vi "__FilterSet_SelfDefine.vi"(8 "error in (no error)":errorcluster, 9 "EIDRef":refnum<vi>[](array[refnum]), 10 "IDRef":refnum<vi>[](array[refnum]), 11 "ControlRef":T1) -> (0 "error out":errorcluster)   [LabVIEW 2011]
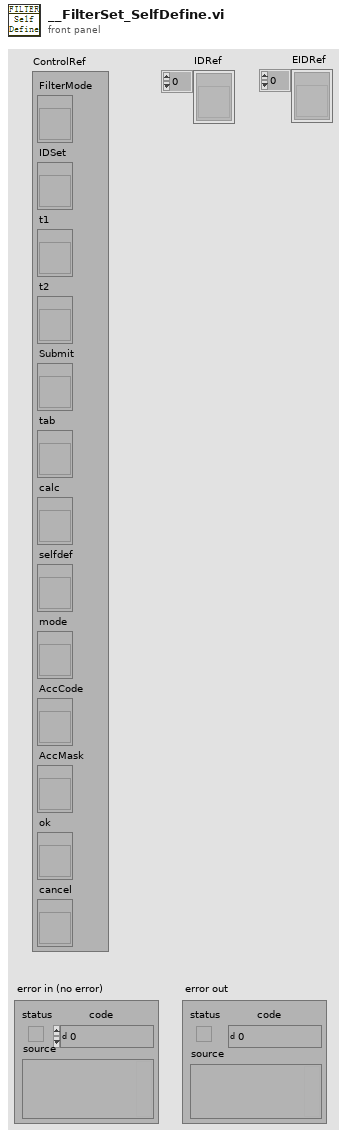
[diagram p1: front panel]
types:
  T1 = cluster{"FilterMode":refnum<vi>, "IDSet":refnum<vi>, "t1":refnum<vi>, "t2":refnum<vi>, "Submit":refnum<vi>, "tab":refnum<vi>, "calc":refnum<vi>, "selfdef":refnum<vi>, "mode":refnum<vi>, "AccCode":refnum<vi>, "AccMask":refnum<vi>, "ok":refnum<vi>, "cancel":refnum<vi>}
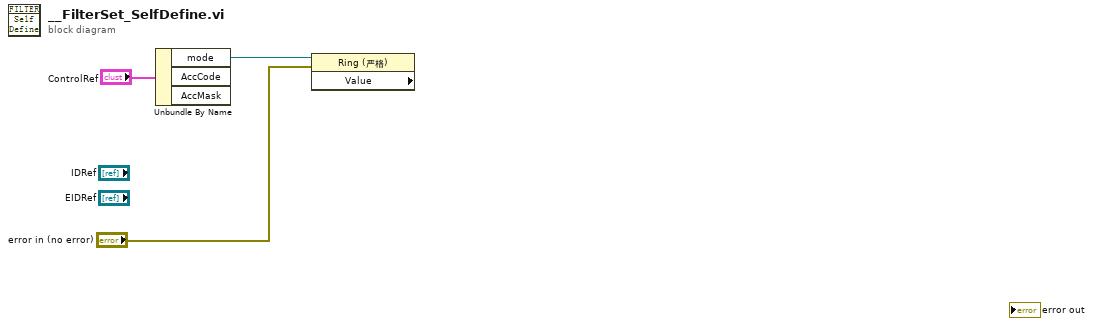
[diagram p0: block diagram]
diagram:
  n1 = Unbundle By Name("ControlRef") -> ("mode"=w2:refnum<vi>)  [unwired: 2 out]
  n2 = property class="Ring (严格)" props=["Value"](reference=w2, error in="error in (no error)") -> ()  [unwired: 3 out]
